vi "Control VI 2.vi"() -> ()   [LabVIEW 2021]
panel:
  in  "DO1.31":bool
  in  "DO1.30":bool
  in  "DO1.29":bool
  in  "DO1.28":bool
  in  "DO1.27":bool
  in  "DO1.26":bool
  in  "DO1.25":bool
  in  "DO1.24":bool
  in  "SOL_Rejection CYL_4":bool
  in  "SOL_Rejection CYL_3":bool
  in  "SOL_Rejection CYL_2":bool
  in  "SOL_Rejection CYL_1":bool
  in  "SOL_Measure_Clamp_CYL":bool
  in  "SOL_Measurement_CYL":bool
  in  "SOL_Insertion_Air_Nozzle":bool
  in  "SOL_Cutting_Clamp_CYL":bool
  in  "SOL_Cutting_CYL":bool
  in  "SOL_Insertion_Clamp_CYL":bool
  in  "SOL_Insertion _CYL":bool
  in  "SOL_Tube_Feed_Gating_CYL":bool
  in  "SOL_Tube_Feed_Agitatator":bool
  in  "SOL_Gating_CYL_Rear":bool
  in  "Pump_CNVR_Motor _ON":bool
  in  "Bowl  Feeder_ ON":bool
  in  "SOL_Index_CNVR_Output _Separator _Rear":bool
  in  "SOL_Index_CNVR_Stopper_Rear":bool
  in  "SOL_Index_CNVR_Rotary_CCW":bool
  in  "SOL_Index_Rotary_CW":bool
  in  "TL_Buzzer":bool
  in  "TL_Green":bool
  in  "TL_Orange":bool
  in  "TL_Red":bool
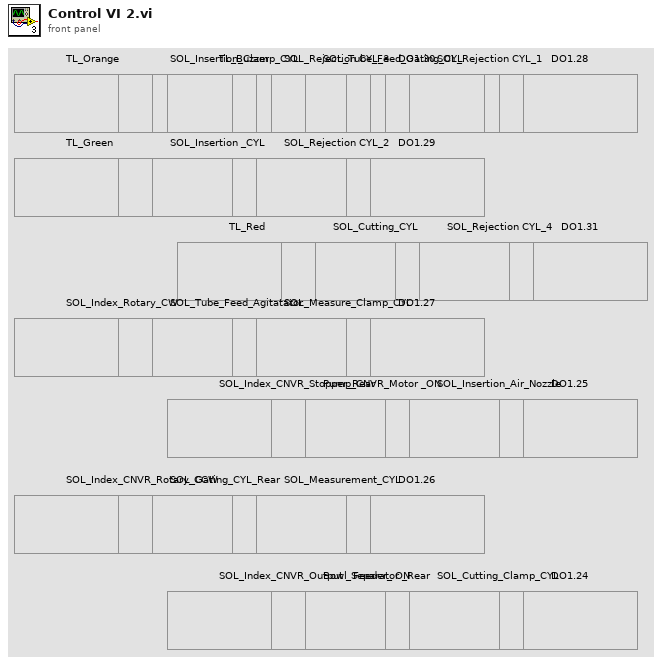
[diagram p1: front panel]
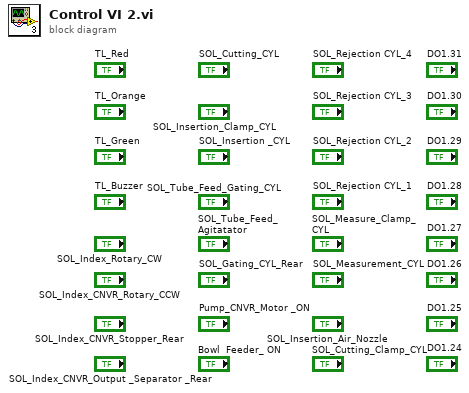
[diagram p0: block diagram]
diagram:
